vi "Read Measurements Menu.vi"(8 "error in (no error)":errorcluster, 11 "Common Measurements Interface in":refnum<class "Common Measurements Interface.lvclass">) -> (0 "error out":errorcluster, 2 "Measurements Menu":refnum<vi>, 3 "Common Measurements Interface out":refnum<class "Common Measurements Interface.lvclass">)   [LabVIEW 2015, in "Common Measurements Interface.lvclass"]
uses:
  Common Measurements Interface.lvclass
  Queued Listbox/Queued Listbox.xctl
  Common Measurements Interface.lvclass/Common Measurements Interface.ctl
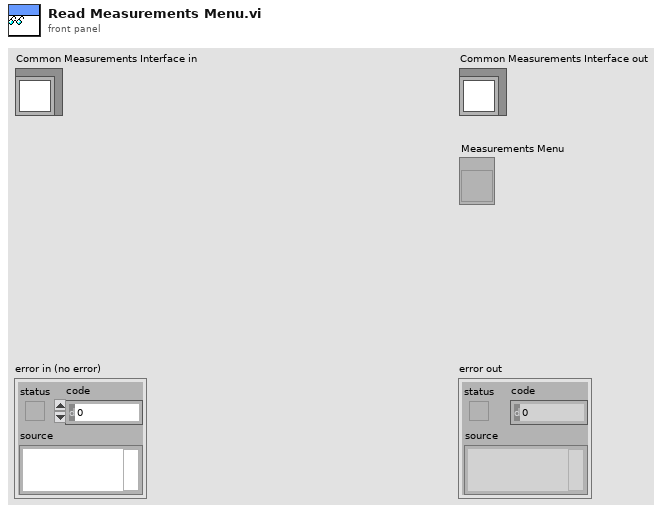
[diagram p1: front panel]
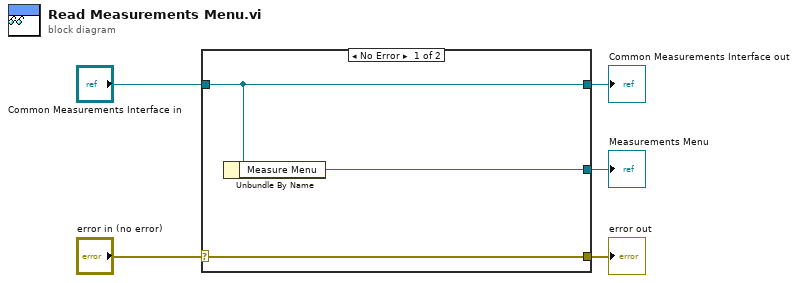
[diagram p0: block diagram]
diagram:
  n1 = case shown="No Error" "error in (no error)" {
    selector: "error in (no error)" -> [w8 w9]
    tunnel: [w8 w9] -> w4
    tunnel: [w7 w10] -> w2
    tunnel: "Common Measurements Interface in" -> [w7 w10]
    tunnel: [w6 _] -> w1
    frame No Error {
      n2 = Unbundle By Name(w7) -> ("Measure Menu"=w6:refnum<vi>)
    }
    frame Error {
    }
  }
  "error out" <- w4
  "Common Measurements Interface out" <- w2
  "Measurements Menu" <- w1
